vi "Error Handler.vi"(8 "error in (no error)":errorcluster, 10 "Error Case":string, 11 "queue in":refnum<queue>) -> (0 "error out":errorcluster, 3 "queue out":refnum<queue>)   [LabVIEW 2012, in "Cmd Queue.lvlib"]
uses:
  Cmd Queue.lvlib
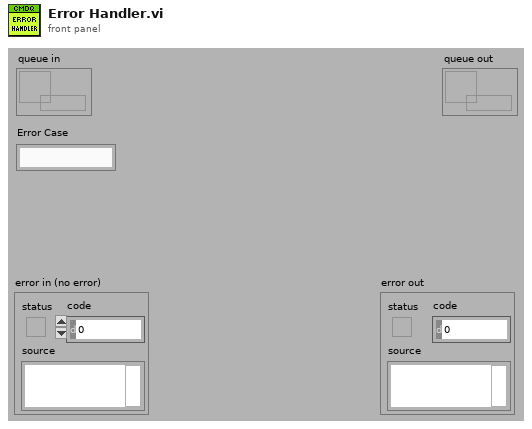
[diagram p1: front panel]
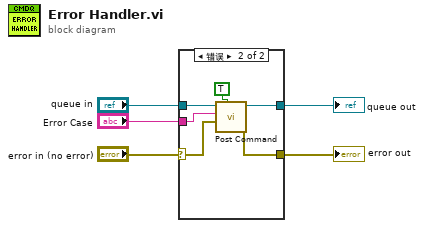
[diagram p0: block diagram]
diagram:
  n1 = case shown="错误" "error in (no error)" {
    selector: "error in (no error)" -> [w6 w8]
    tunnel: "queue in" -> [w7 w13]
    tunnel: [w7 w12] -> w4
    tunnel: "Error Case" -> [_ w11]
    tunnel: [w6 w9] -> w1
    frame No Error {
    }
    frame Error {
      n2 = call "Post Command.vi"("Priority?"=TRUE, "Data"=w8, "Command"=w11, "queue in"=w13) -> ("error out"=w9:errorcluster, "queue out"=w12:refnum<queue>)  [unwired: 5 in, 1 out]
    }
  }
  "error out" <- w1
  "queue out" <- w4
